vi "Close.vi"(8 "error in (no error)":errorcluster, 10 "Flush stream":bool, 11 "NetworkStreamWriter in":refnum<class "NetworkStreamWriter.lvclass">) -> (0 "error out":errorcluster, 3 "NetworkStreamWriter out":refnum<class "NetworkStreamWriter.lvclass">)   [LabVIEW 2011, in "NetworkStreamWriter.lvclass"]
doc: "This VI closes references internal to the NetworkStreamWriter object. This allows memory to be cleaned up effectively."
uses:
  NetworkStreamWriter.lvclass
  NetworkStreamWriter.lvclass/NetworkStreamWriter.ctl
  <vilib>/dex/Flush And Wait Empty Condition.ctl
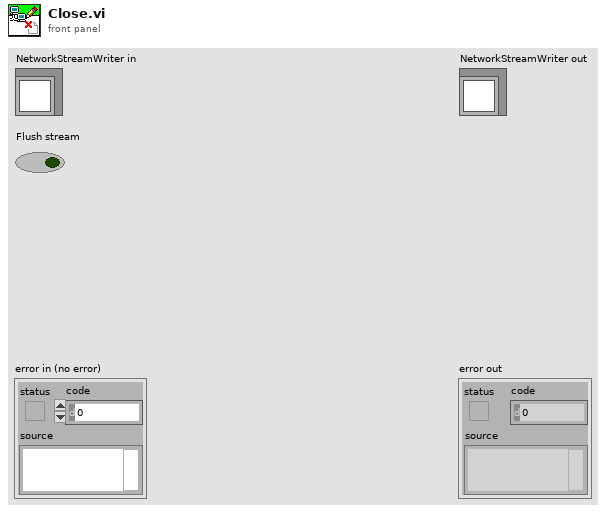
[diagram p1: front panel]
types:
  T1 = typedef "Flush And Wait Empty Condition.ctl" = u8
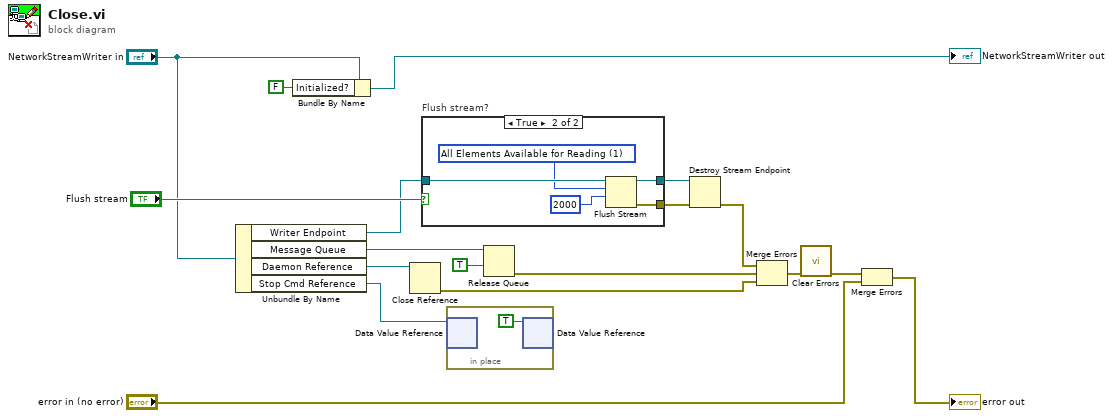
[diagram p0: block diagram]
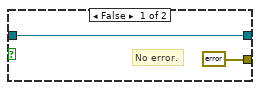
[diagram p2: hidden frame]
diagram:
  n1 = Unbundle By Name("NetworkStreamWriter in") -> ("Writer Endpoint"=w11:refnum<k21>, "Message Queue"=w16:refnum<queue>, "Daemon Reference"=w17:refnum<vi>, "Stop Cmd Reference"=w14:refnum<data-value>)
  n2 = Bundle By Name(cluster="NetworkStreamWriter in", "Initialized?"=FALSE) -> (→"NetworkStreamWriter out":refnum<class "NetworkStreamWriter.lvclass">)
  n3 = Close Reference(reference=w17) -> (error out=w5:errorcluster)  [unwired: 1 in]
  n4 = case "Flush stream?" shown="True" "Flush stream" {
    tunnel: w11 -> [w20 w25]
    tunnel: [w20 w24] -> w10
    tunnel: [errorcluster {"status"=FALSE, "code"=0, "source"=""} ("error out") w23] -> w9
    frame False {
      # "No error."
    }
    frame True {
      w22 = T1 1 items=["All Elements Read From Stream", "All Elements Available for Reading"] ("wait condition")
      n5 = Flush Stream(9:2000 ("timeout in ms (-1)"), 10:w22, 11:w25) -> (0:w23:errorcluster, 3:w24:refnum<k21>)  [unwired: 1 in, 1 out]
    }
  }
  n6 = in-place {
    n7 = in-place-dvr #1(w14) -> ()  [unwired: 2 out]
    n8 = in-place-dvr #1(TRUE ("data value")) -> ()  [unwired: 2 out]
  }
  n9 = Release Queue(queue=w16, force destroy? (F)=TRUE) -> (error out=w12:errorcluster)  [unwired: 1 in, 2 out]
  n10 = Destroy Stream Endpoint(8:w9, 11:w10) -> (0:w13:errorcluster)
  n11 = Merge Errors(w13, w12, w5) -> (w4:errorcluster)
  n12 = call <vilib>:"Clear Errors.vi"("error in (no error)"=w4) -> ("error out"=w3:errorcluster)  [unwired: 6 in]
  n13 = Merge Errors(w3, "error in (no error)") -> (→"error out":errorcluster)
